vi "Run.vi"(8 "error in (no error)":errorcluster, 9 "s on last turn":dbl, 10 "Maze (0: Empty, -1: Enemy. >0: Teammate":i32[][](array[numeric]), 11 "Attack in":refnum<class "Spread.lvclass">) -> (0 "error out":errorcluster, 1 "Direction":T1, 2 "Action":T2, 3 "Attack out":refnum<class "Spread.lvclass">, 4 "Replicated":refnum<class "Square.lvclass">)   [LabVIEW 2015, in "Spread.lvclass"]
uses:
  Spread.lvclass
  Type Defs/Action Enum.ctl
  Type Defs/Direction Enum.ctl
  Square/Square.lvclass
  Spread.lvclass/Spread.ctl
  Write Direction.vi
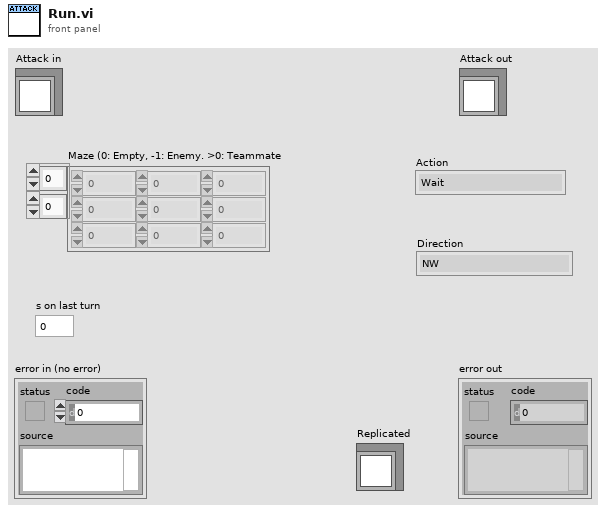
[diagram p1: front panel]
types:
  T1 = typedef "Square.lvclass/Direction Enum.ctl" = enum16{"NW", "N", "NE", "E", "SE", "S", "SW", "W"}
  T2 = typedef "Square.lvclass/Action Enum.ctl" = enum16{"Wait", "Move", "Attack", "Replicate"}
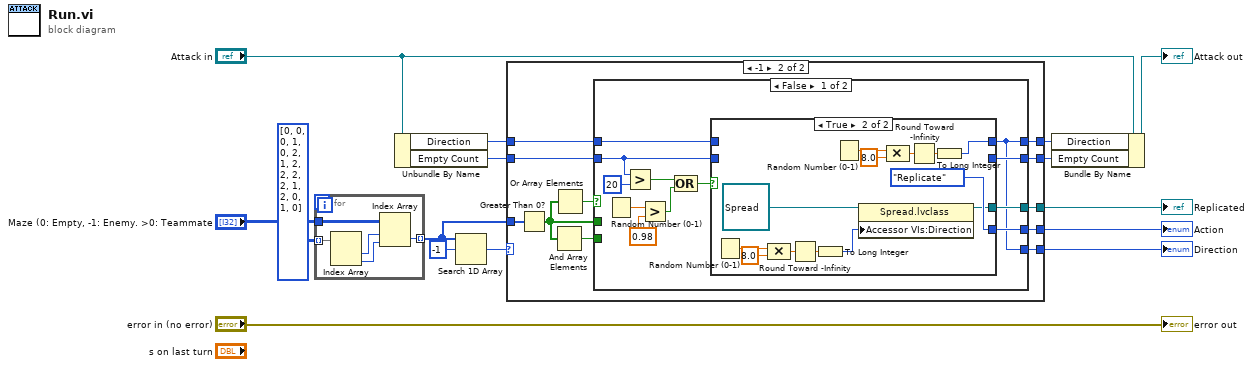
[diagram p0: block diagram]
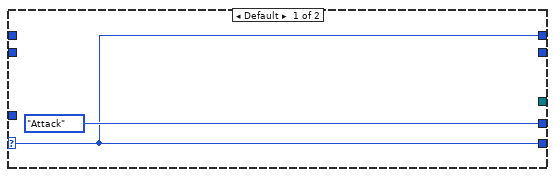
[diagram p2: hidden frame]
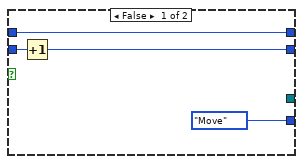
[diagram p3: hidden frame]
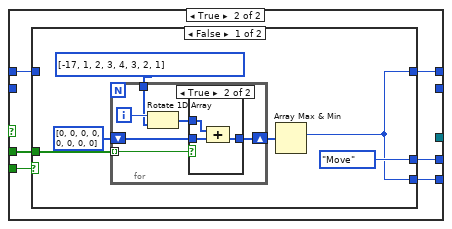
[diagram p4: hidden frame]
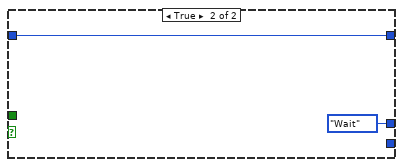
[diagram p6: hidden frame]
diagram:
  n1 = for {
    tunnel: "Maze (0: Empty, -1: Enemy. >0: Teammate" -> [w20]
    tunnel: i32[][] [[0, 0], [0, 1], [0, 2], [1, 2], [2, 2], [2, 1], [2, 0], [1, 0]] -> [w19] mode=indexing
    tunnel: [w16] -> w8 mode=indexing
    n2 = Index Array(array=w19) -> (element #1=w18:i32, element #2=w17:i32)  [unwired: 2 in]
    n3 = Index Array(array=w20, index (row)=w18, index (col)=w17) -> (element=w16:i32)
  }
  n4 = Unbundle By Name("Attack in") -> ("Direction"=w6:T1, "Empty Count"=w7:i32)
  n5 = Search 1D Array(1D array=w8, element=-1) -> (index of element=w9:i32)  [unwired: 1 in]
  n6 = case shown="-1" w9 {
    selector: w9 -> [w21 _]
    tunnel: [w21 w30] -> w2
    tunnel: [Action_Enum."Attack" ("Action") w29] -> w3
    tunnel: w6 -> [_ w32]
    tunnel: w8 -> [_ w33]
    tunnel: [w21 w31] -> w1
    tunnel: w7 -> [_ w26]
    tunnel: [_ w25] -> w5
    tunnel: [_ w24] -> w4
    frame Default {
    }
    frame -1 {
      n7 = Greater Than 0?(x=w33) -> (x > 0?=w28:bool[])
      n8 = And Array Elements(Boolean array=w28) -> (logical AND=w27:bool)
      n9 = Or Array Elements(Boolean array=w28) -> (logical OR=w23:bool)
      n10 = case shown="False" w23 {
        tunnel: w32 -> [w35 w63]
        tunnel: [w34 w64] -> w31
        tunnel: [w34 w66] -> w30
        tunnel: [w45 w68] -> w29
        tunnel: w28 -> [_ w67]
        tunnel: w27 -> [_ w65]
        tunnel: w26 -> [w36 _]
        tunnel: [w44 _] -> w25
        tunnel: [w43 _] -> w24
        frame False {
          n11 = Random Number (0-1)() -> (number: 0 to 1=w40:dbl)
          n12 = Greater?(x=w36, y=20) -> (0:w41:bool)
          n13 = Greater?(x=w40, y=0.98) -> (0:w38:bool)
          n14 = Compound Arithmetic op=OR(w41, w38) -> (w37:bool)
          n15 = case shown="True" w37 {
            tunnel: [Action_Enum."Move" ("t") Action_Enum."Replicate" ("t")] -> w45
            tunnel: [w48 _] -> w44
            tunnel: [_ w61] -> w43
            tunnel: w36 -> [w47 _]
            tunnel: w35 -> [w46 _]
            tunnel: [w46 w50] -> w34
            frame False {
              n16 = Increment(x=w47) -> (x+1=w48:i32)
            }
            frame True {
              n17 = Random Number (0-1)() -> (number: 0 to 1=w59:dbl)
              n18 = Compound Arithmetic op=MULTIPLY(w59, 8.0 ("value")) -> (w57:dbl)
              n19 = Round Toward -Infinity(1:w57) -> (0:w56:dbl)
              n20 = To Long Integer(number=w56) -> (32bit integer=w55:i32)
              n21 = Random Number (0-1)() -> (number: 0 to 1=w51:dbl)
              n22 = property class="Spread.lvclass"(reference=refnum<class "Spread.lvclass"> refnum ("Spread.lvclass"), "Accessor VIs:Direction"=w55) -> (reference out=w61:refnum<class "Spread.lvclass">)  [unwired: 1 in, 1 out]
              n23 = Compound Arithmetic op=MULTIPLY(w51, 8.0 ("value")) -> (w53:dbl)
              n24 = Round Toward -Infinity(1:w53) -> (0:w54:dbl)
              n25 = To Long Integer(number=w54) -> (32bit integer=w50:i32)
            }
          }
        }
        frame True {
          n26 = case shown="False" w65 {
            tunnel: [Action_Enum."Move" ("Action") Action_Enum."Wait" ("Action")] -> w68
            tunnel: w67 -> [w73 _]
            tunnel: [w69 _] -> w66
            tunnel: [w69 w86] -> w64
            tunnel: w63 -> [_ w86]
            frame False {
              n27 = for {
                tunnel: w73 -> [w78] mode=indexing
                tunnel: i32[] [-17, 1, 2, 3, 4, 3, 2, 1] -> [w79]
                shift-right: [w76] -> w70
                shift-left: i32[] [0, 0, 0, 0, 0, 0, 0, 0] -> [w75]
                i -> [w80]
                n28 = Rotate 1D Array(1:w79, 2:w80) -> (0:w77:i32[])
                n29 = case shown="True" w78 {
                  tunnel: w77 -> [_ w84]
                  tunnel: [w81 w83] -> w76
                  tunnel: w75 -> [w81 w82]
                  frame False {
                  }
                  frame True {
                    n30 = Compound Arithmetic op=ADD(w84, w82) -> (w83:i32[])
                  }
                }
              }
              n31 = Array Max & Min(array=w70) -> (max index (indices)=w69:i32)  [unwired: 3 out]
            }
            frame True {
            }
          }
        }
      }
    }
  }
  "Action" <- w3
  "Direction" <- w2
  "Replicated" <- w4
  n32 = Bundle By Name(cluster="Attack in", "Direction"=w1, "Empty Count"=w5) -> (→"Attack out":refnum<class "Spread.lvclass">)
  "error out" <- "error in (no error)"
